vi "Save out values and integrate at the end of measurementJJCH2 (SubVI).vi"(4 "Measurement Array":dbl[](array[numeric]), 5 "Path":path, 6 "Time Array":dbl[](array[numeric]), 8 "ListBox in 2":refnum<vi>, 9 "Integrate Array":dbl[](array[numeric]), 10 "Measurement running?":bool, 11 "XYGraph Refnum":refnum<vi>) -> (0 "?":cluster{"all rows":dbl[], "all rows":dbl[]}(graph), 1 "Concentrations":dbl[](array[numeric]), 2 "element":string, 3 "size(s)":i32)   [LabVIEW 2014]
panel:
  out "error out":errorcluster
  out "Lac concentration":dbl format="%.4f"
  out "Xyl concentration":dbl format="%.4f"
  out "Glu concentration":dbl format="%.4f"
  out "Lac area":dbl format="%.6e"
  out "Xyl area":dbl format="%.6e"
  out "Glu area":dbl format="%.6e"
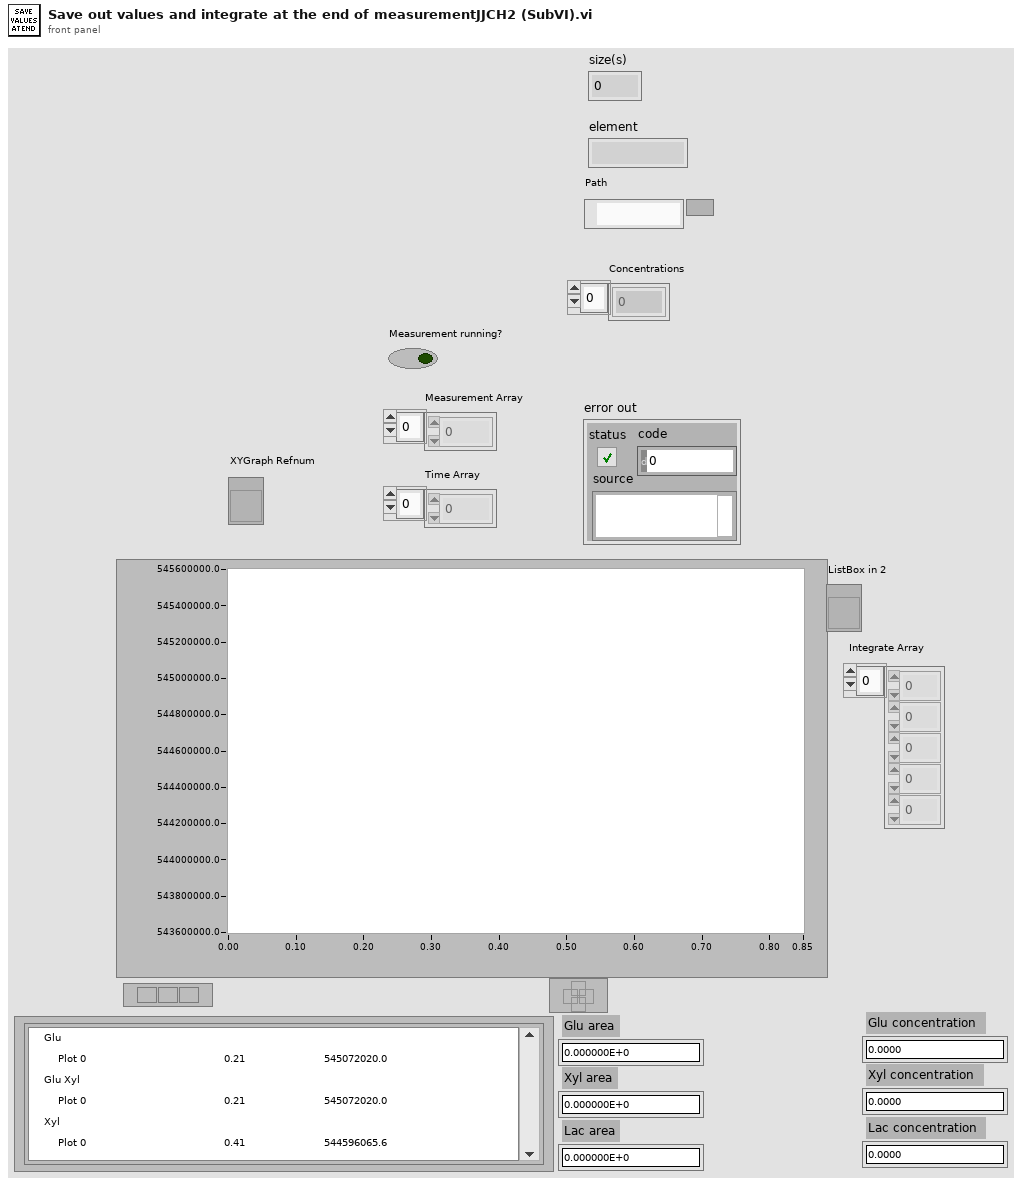
[diagram p1: front panel]
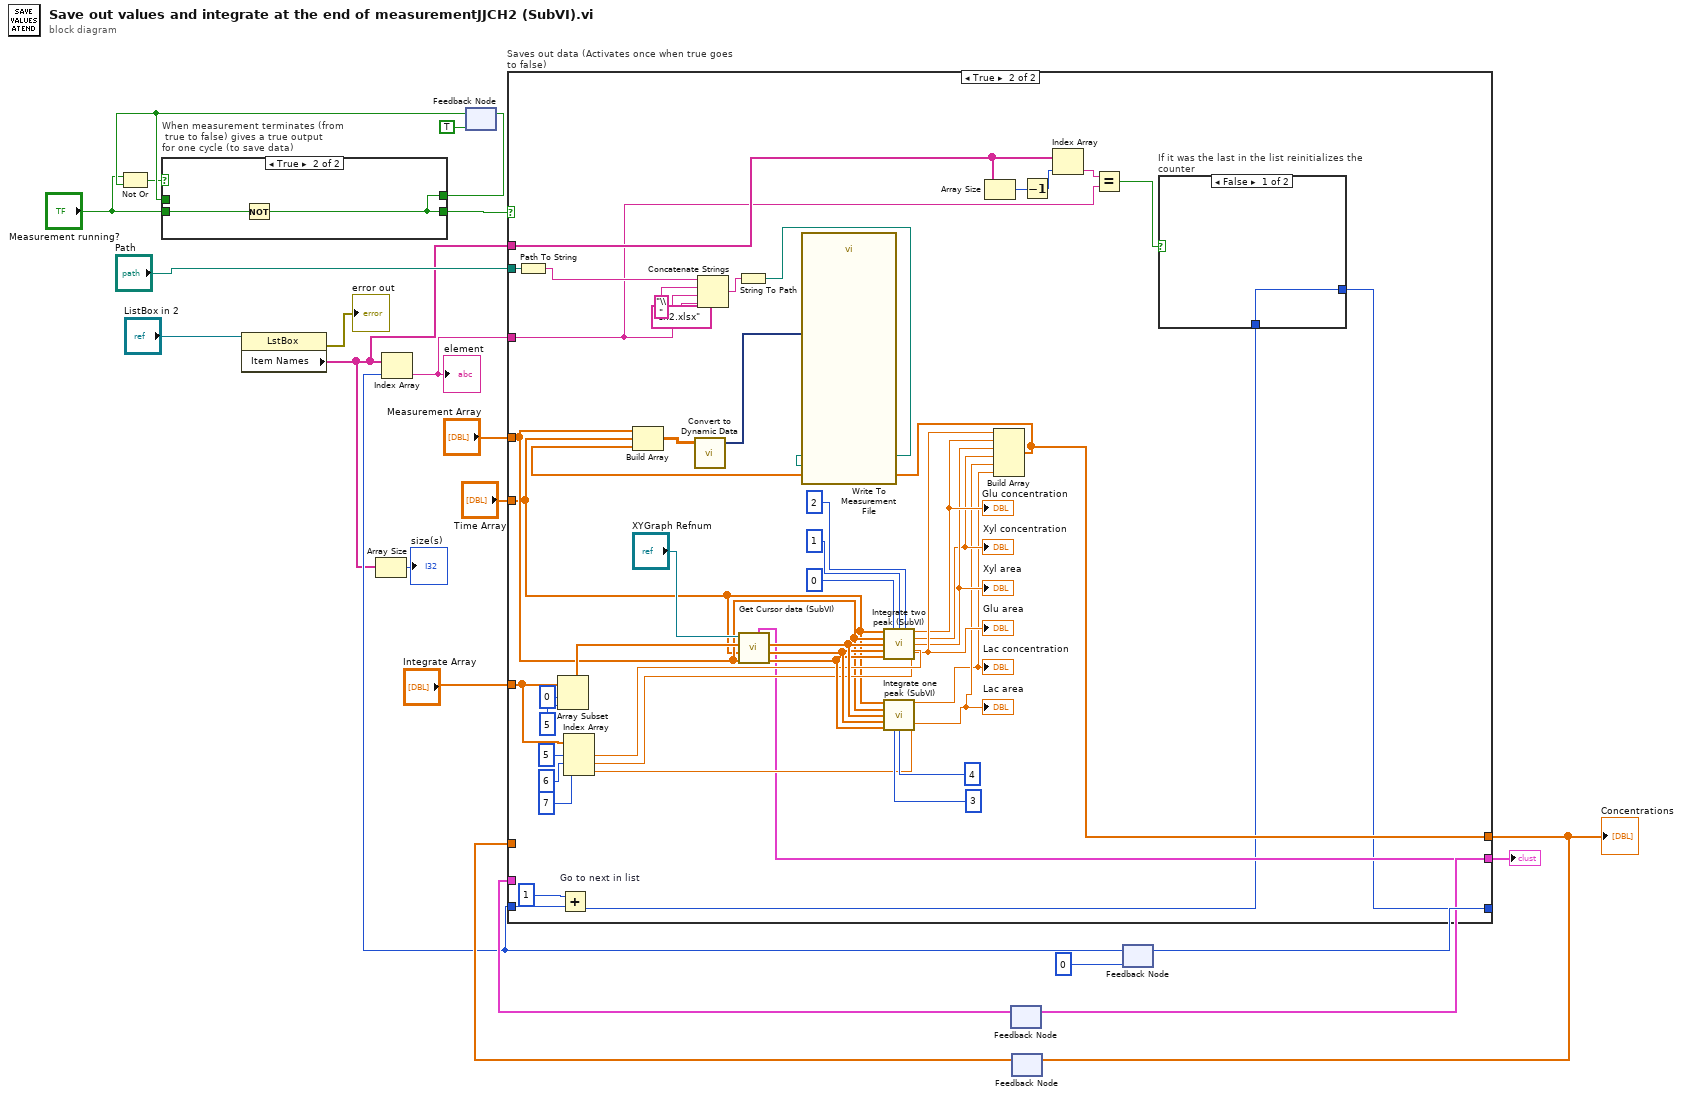
[diagram p0: block diagram]
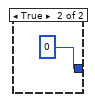
[diagram p3: hidden frame]
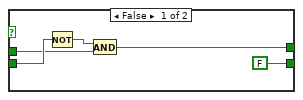
[diagram p4: hidden frame]
diagram:
  n1 = property on="Property Node" class="LstBox"(reference="ListBox in 2") -> (error out=→"error out":errorcluster, "Item Names"=w1:string[])  [unwired: 1 in, 1 out]
  n2 = Array Size(array=w1) -> (size(s)=→"size(s)":i32)
  n3 = feedback #1(TRUE) -> (w19:bool)
  n4 = Not Or(1:w19, 2:"Measurement running?") -> (0:w16:bool)
  n5 = case "When measurement terminates (from\n true to false) gives a true output \nfor one cycle (to save data)" shown="True" w16 {
    tunnel: "Measurement running?" -> [w27 w29]
    tunnel: [w26 w28] -> w14
    tunnel: w19 -> [w23 _]
    tunnel: [FALSE w28] -> w15
    frame False {
      n6 = Not(x=w27) -> (.not. x?=w24:bool)
      n7 = And(x=w24, y=w23) -> (x .and. y?=w26:bool)
    }
    frame True {
      n8 = Not(x=w29) -> (.not. x?=w28:bool)
    }
  }
  n9 = feedback-in #1(w14) -> ()
  n10 = feedback #2() -> (w5:cluster{"all rows":dbl[], "all rows":dbl[]})  [unwired: 1 in]
  n11 = feedback #3() -> (w4:dbl[])  [unwired: 1 in]
  n12 = feedback #4(0) -> (w2:i32)
  n13 = Index Array(array=w1, index=w2) -> (element=w12:string)
  "element" <- w12
  n14 = case "Saves out data (Activates once when true goes to false)" shown="True" w15 {
    tunnel: [w32 w35] -> w10
    tunnel: w2 -> [w32 w75]
    tunnel: "Measurement Array" -> [_ w42]
    tunnel: "Time Array" -> [_ w41]
    tunnel: "Path" -> [_ w77]
    tunnel: w12 -> [_ w39]
    tunnel: "Integrate Array" -> [_ w61]
    tunnel: [w31 w47] -> w6
    tunnel: w5 -> [w31 _]
    tunnel: [w30 w46] -> w3
    tunnel: w4 -> [w30 _]
    tunnel: w1 -> [_ w40]
    frame False {
    }
    frame True {
      n15 = Path To String(path=w77) -> (string=w43:string)
      n16 = Array Subset(array=w61, index=0, length=5) -> (w62:dbl[])
      n17 = Add "Go to next in list"(x=1, y=w75) -> (x+y=w36:i32)
      n18 = Index Array(array=w61, index #1=5 ("index"), index #2=6 ("index"), index #3=7 ("index")) -> (element #1=w57:dbl, element #2=w56:dbl, element #3=w55:dbl)
      n19 = Concatenate Strings(w43, "\\" ("string"), w39, "ch2.xlsx" ("string")) -> (w44:string)
      n20 = String To Path(string=w44) -> (path=w45:path)
      n21 = call "Get Cursor data (SubVI).vi"("Signal"=w42, "Time"=w41, "Time position"=w62, "XYGraph Refnum"="XYGraph Refnum") -> ("Signal cursor"=w68:dbl[], "Time cursor"=w69:dbl[], "Index cursor"=w70:dbl[], 5:w47:cluster{"all rows":dbl[], "all rows":dbl[]})  [unwired: 4 in]
      n22 = call "Integrate two peak (SubVI).vi"("Time array"=w41, "Start cursor index"=0 ("index"), "Separator cursor index"=1 ("index"), "End cursor index"=2 ("index"), "Signal array"=w42, "Index cursor"=w70, "Time cursor"=w69, "Glu standard area"=w57, "Signal cursor"=w68, "Xyl standard area"=w56) -> ("Glu concentration"=w53:dbl, "Xyl concentration"=w51:dbl, "Glu area"=w54:dbl, "Xyl area"=w52:dbl)  [unwired: 2 in]
      "Glu area" <- w54
      "Xyl area" <- w52
      "Glu concentration" <- w53
      "Xyl concentration" <- w51
      n23 = call "Integrate one peak (SubVI).vi"("Time array"=w41, "Start Index"=3 ("index"), "End Index"=4 ("index"), "Signal Array"=w42, "Index cursor"=w70, "Time cursor"=w69, "Signal cursor"=w68, "Lac standard area"=w55) -> ("Lac concentration"=w49:dbl, "Lac area"=w50:dbl)  [unwired: 6 in]
      "Lac area" <- w50
      "Lac concentration" <- w49
      n24 = Array Size(array=w40) -> (size(s)=w34:i32)
      n25 = Build Array(w54, w53, w52, w51, w50, w49) -> (w46:dbl[])
      n26 = Build Array(w42, w41, w46) -> (w79:dbl[][])
      n27 = call "Convert to Dynamic Data"("2D Array"=w79) -> ("Dynamic Data Type"=w78:dynamicdata)  [unwired: 3 in]
      n28 = call "Write To Measurement File"("Signals"=w78, "Filename"=w45) -> ()  [unwired: 15 in, 3 out]
      n29 = Decrement(x=w34) -> (x-1=w33:i32)
      n30 = Index Array(array=w40, index=w33) -> (element=w38:string)
      n31 = Equal?(x=w38, y=w39) -> (x = y?=w37:bool)
      n32 = case "If it was the last in the list reinitializes the counter" shown="False" w37 {
        tunnel: w36 -> [w80 _]
        tunnel: [w80 0] -> w35
        frame False {
        }
        frame True {
        }
      }
    }
  }
  "?" <- w6
  "Concentrations" <- w3
  n33 = feedback-in #2(w6) -> ()
  n34 = feedback-in #3(w3) -> ()
  n35 = feedback-in #4(w10) -> ()
